vi "Create 2D Array Pointer.vi"(8 "error in (no error)":errorcluster, 10 "size Dim 2":u32, 11 "size Dim 1":u32) -> (0 "error out":errorcluster, 3 "Pointer":u64)   [LabVIEW 2017, in "MU_3SL_interface.lvlib"]
uses:
  MU_3SL_interface.lvlib
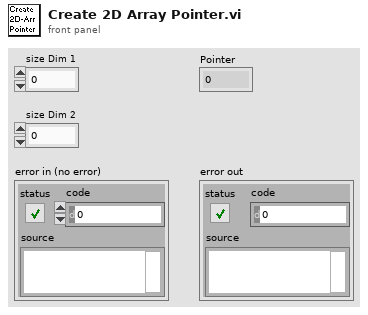
[diagram p1: front panel]
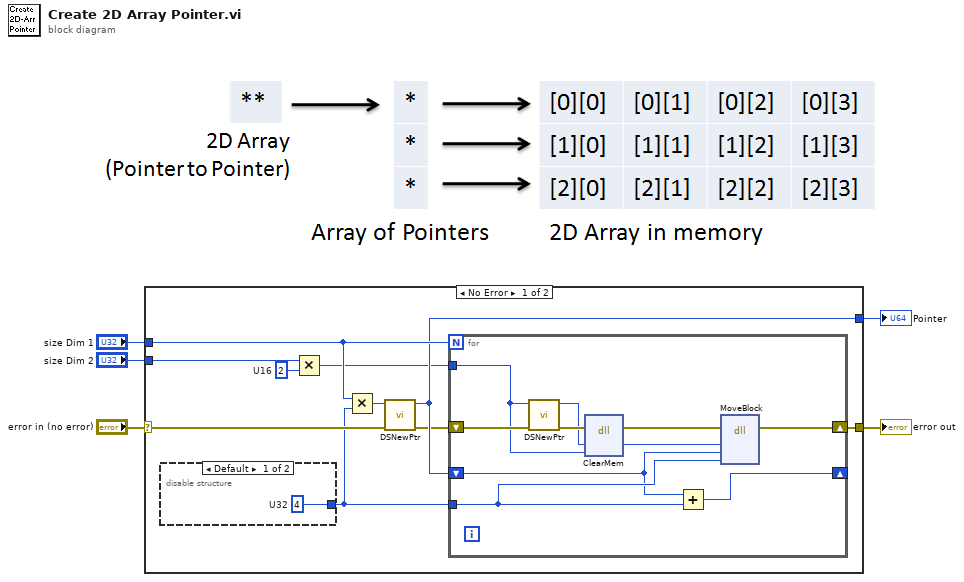
[diagram p0: block diagram]
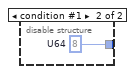
[diagram p2: hidden frame]
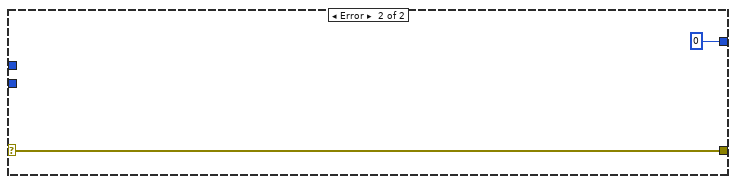
[diagram p3: hidden frame]
diagram:
  n1 = case shown="No Error" "error in (no error)" {
    selector: "error in (no error)" -> [w11 w29]
    tunnel: "size Dim 2" -> [w15 _]
    tunnel: "size Dim 1" -> [w14 _]
    tunnel: [w13 w29] -> w3
    tunnel: [w12 u64 0 ("Pointer")] -> w2
    frame No Error {
      w10 = u32 2  # U16
      n2 = disable-structure shown="Default" {
        disable-tunnel: [w16 w17] -> w6
        frame condition #0 (active) {
          w16 = u32 4  # U32
        }
        frame condition #1 {
          w17 = u64 8  # U64
        }
      }
      n3 = Multiply(x=w15, y=w10) -> (x*y=w9:u32)
      n4 = Multiply(x=w14, y=w6) -> (x*y=w7:u32)
      n5 = call <vilib>:"DSNewPtr.vi"("error in (no error)"=w11, "Size"=w7) -> ("error out"=w8:errorcluster, "Pointer"=w12:u64)  [unwired: 8 in]
      n6 = for {
        N: w14 -> [_]
        tunnel: w9 -> [w25]
        shift-right: [w19] -> w13
        shift-left: w8 -> [w27]
        tunnel: w6 -> [w22]
        shift-right: [w20] -> _
        shift-left: w12 -> [w21]
        n7 = call <vilib>:"DSNewPtr.vi"("error in (no error)"=w27, "Size"=w25) -> ("error out"=w26:errorcluster, "Pointer"=w18:u64)  [unwired: 8 in]
        n8 = dll-call lib="LabVIEW" fn="ClearMem"(error in=w26, "pointer"=w18, "size"=w25) -> (error out=w24:errorcluster, "pointer"=w23:i64)  [unwired: 4 in, 1 out]
        n9 = Add(x=w21, y=w22) -> (x+y=w20:u64)
        n10 = dll-call lib="LabVIEW" fn="MoveBlock"(error in=w24, "source"=w23, "dest"=w21, "size"=w22) -> (error out=w19:errorcluster)  [unwired: 6 in, 1 out]
      }
    }
    frame Error {
    }
  }
  "error out" <- w3
  "Pointer" <- w2
